vi "Write Recording pulse.vi"(8 "error in (no error)":errorcluster, 10 "Armed":bool=TRUE, 11 "Pulse Driver in":refnum<class "Pulse Driver.lvclass">) -> (0 "error out":errorcluster, 3 "Pulse Driver out":refnum<class "Pulse Driver.lvclass">)   [LabVIEW 2021, in "Pulse Driver.lvclass"]
uses:
  Pulse Driver.lvclass
  Pulse Driver.lvclass/Pulse Driver.ctl
panel:
  out "Array - String":string[](array[string])
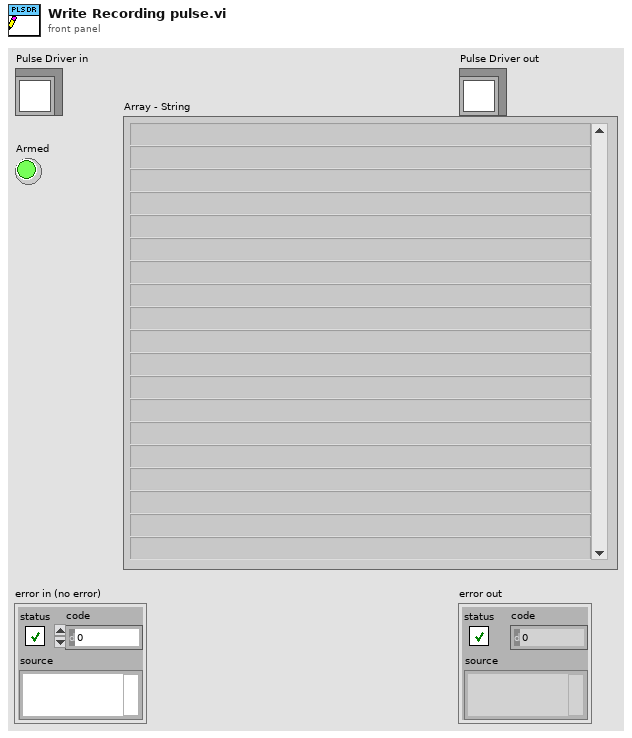
[diagram p1: front panel]
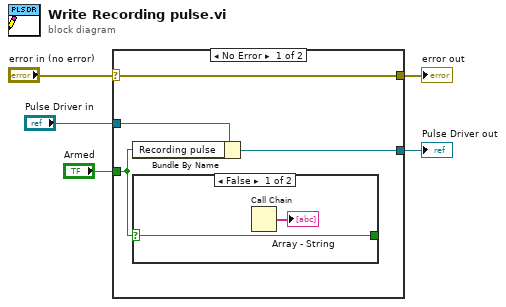
[diagram p0: block diagram]
diagram:
  n1 = case shown="No Error" "error in (no error)" {
    selector: "error in (no error)" -> [w9 w13]
    tunnel: [w9 w13] -> w4
    tunnel: [w7 w14] -> w2
    tunnel: "Pulse Driver in" -> [w8 w14]
    tunnel: "Armed" -> [w6 _]
    frame No Error {
      n2 = Bundle By Name(cluster=w8, "Recording pulse"=w6) -> (w7:refnum<class "Pulse Driver.lvclass">)
      n3 = case shown="False" w6 {
        selector: w6 -> [w11 w12]
        tunnel: [w11 w12] -> _
        frame False {
          n4 = Call Chain() -> (call chain=→"Array - String":string[])
        }
        frame True {
        }
      }
    }
    frame Error {
    }
  }
  "error out" <- w4
  "Pulse Driver out" <- w2
